vi "Read Pressure DBL.vi"(8 "error in":errorcluster, 10 "Source":string, 11 "Virtual NEO480 in":refnum<class "Virtual NEO480.lvclass">) -> (0 "error out":errorcluster, 1 "Time Stamp":timestamp format="%<%x %.3X>T", 2 "Pressure":dbl, 3 "Virtual NEO480 out":refnum<class "Virtual NEO480.lvclass">)   [LabVIEW 2024, in "Virtual NEO480.lvclass"]
uses:
  Virtual NEO480.lvclass
  D:/git/HAL/Source/Action Point/Action Point.lvclass
  Source/Action Point/Action Point.lvclass/Action Point.ctl
  Virtual NEO480.lvclass/Virtual NEO480.ctl
  Source/Interfaces/ILog Data/ILog Data.lvclass
  Source/DBC Communicator/DBC Communicator.lvclass
  Source/Action Point/Action Point.lvclass
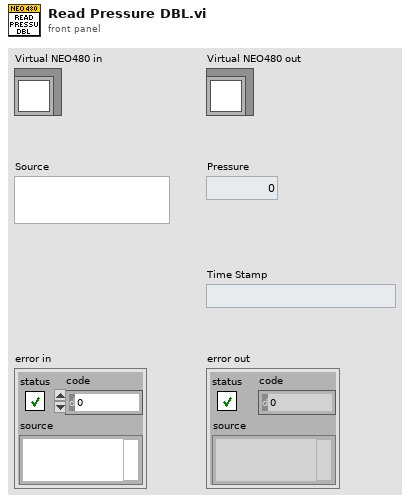
[diagram p1: front panel]
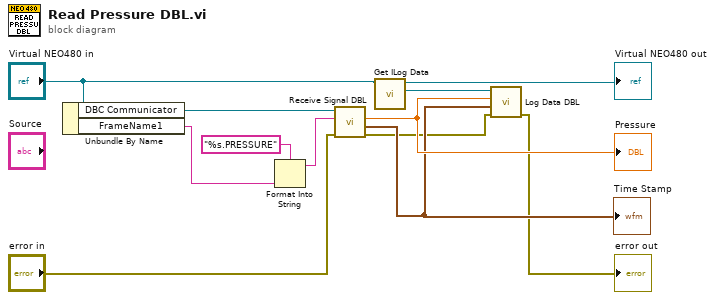
[diagram p0: block diagram]
diagram:
  n1 = Unbundle By Name("Virtual NEO480 in") -> ("DBC Communicator"=w12:refnum<class "DBC Communicator.lvclass">, "FrameName1"=w10:string)
  n2 = Format Into String(format string="%s.PRESSURE", w10) -> (resulting string=w9:string)  [unwired: 2 in, 1 out]
  n3 = call "Receive Signal DBL.vi"("error in"="error in", "Signal Name"=w9, "DBC Communication in"=w12) -> ("error out"=w2:errorcluster, "Time Stamp"=w3:timestamp, "Value"=w4:dbl)  [unwired: 5 in, 1 out]
  "Pressure" <- w4
  "Time Stamp" <- w3
  n4 = call "Get ILog Data.vi"("Action Point in"="Virtual NEO480 in") -> ("ILog Data"=w7:refnum<class "ILog Data.lvclass">, "Action Point out"=→"Virtual NEO480 out":refnum<class "Virtual NEO480.lvclass">)  [unwired: 9 in]
  n5 = call-dynamic "Log Data DBL.vi"("error in"=w2, "Time Stamp"=w3, "Data"=w4, "IDataLogger in"=w7) -> ("error out"=→"error out":errorcluster)  [unwired: 6 in, 1 out]
